vi "TeclaPresionada.vi"(11 "Keyboard":bool[][](array[boolean])) -> (3 "Numeric":dbl)   [LabVIEW 2020]
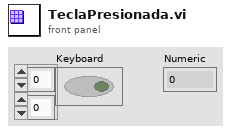
[diagram p1: front panel]
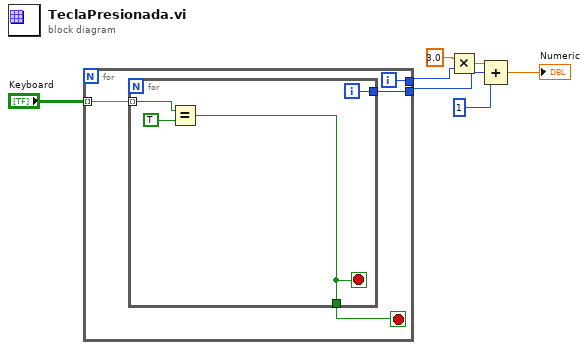
[diagram p0: block diagram]
diagram:
  n1 = for {
    tunnel: "Keyboard" -> [w11] mode=indexing
    tunnel: [w9] -> w2
    tunnel: [w8] -> w7
    i -> [w8]
    stop <- w10 stop-if-true
    n2 = for {
      tunnel: w11 -> [w15] mode=indexing
      tunnel: [w13] -> w10
      tunnel: [w12] -> w9
      i -> [w12]
      stop <- w13 stop-if-true
      n3 = Equal?(x=w15, y=TRUE) -> (x = y?=w13:bool)
    }
  }
  n4 = Multiply(x=3.0, y=w7) -> (x*y=w5:dbl)
  n5 = Compound Arithmetic op=ADD(w5, w2, 1 ("value")) -> (→"Numeric":dbl)
